vi "fetch from db.vi"(8 "error in (no error)":errorcluster, 10 "istruzione select from":string, 11 "Refnum in":T1) -> (3 "data":string[][](array[string]))   [LabVIEW 2016]
uses:
  <vilib>/addons/database/Connection.llb/Conn ObjectReference.ctl
  <vilib>/addons/database/Connection.llb/Conn Execute.vi
  <vilib>/addons/database/Recordset.llb/Rec Fetch Recordset Data (R).vi
  <vilib>/addons/database/Recordset.llb/Rec Destroy - Connection.vi
  <vilib>/addons/database/_DB Variant To Data/Database Variant To Data.xnode
  <vilib>/addons/database/NI_Database_API.lvlib
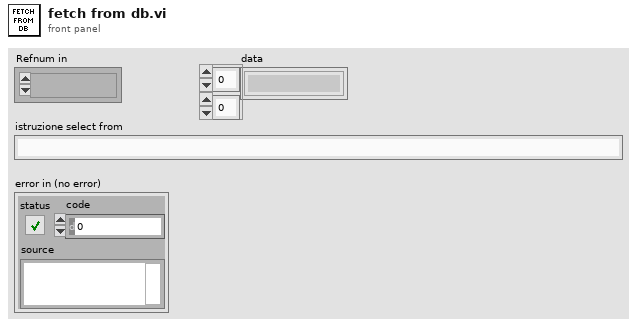
[diagram p1: front panel]
types:
  T1 = typedef "NI_Database_API.lvlib/Conn ObjectReference.ctl" = refnum<k1>
  T2 = typedef "NI_Database_API.lvlib/Rec ObjectReference.ctl" = refnum<k1>
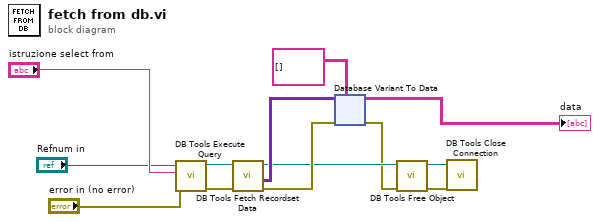
[diagram p0: block diagram]
diagram:
  n1 = call-poly <vilib>:"DB Tools Execute Query.vi"("error in (no error)"="error in (no error)", "SQL query"="istruzione select from", "connection reference"="Refnum in") -> ("error out"=w11:errorcluster, "recordset reference"=w10:T2)  [unwired: 5 in]
  n2 = call-poly <vilib>:"DB Tools Fetch Recordset Data.vi"("error in (no error)"=w11, "recordset reference"=w10) -> ("error out"=w7:errorcluster, "recordset data"=w9:variant[][], "recordset reference out"=w5:T2)  [unwired: 3 in]
  n3 = xnode "Database Variant To Data"("database variant"=w9, "error in"=w7, "type"=string[][] []) -> ("data"=→"data":string[][], "error out"=w4:errorcluster)
  n4 = call-poly <vilib>:"DB Tools Free Object.vi"("error in (no error)"=w4, "recordset reference"=w5) -> ("error out"=w2:errorcluster, "connection reference"=w3:T1)  [unwired: 8 in]
  n5 = call <vilib>:"DB Tools Close Connection.vi"("error in (no error)"=w2, "connection reference"=w3) -> ()  [unwired: 5 in, 1 out]
